vi "loop_config.vi"() -> ()   [LabVIEW 2017]
panel:
  in  "stop":bool
  out "error out":errorcluster
  in  "Read (TRUE)":bool
  in  "In":u8=22 format="%.0x"
  in  "Address":u32=2305 format="%x"
  out "Out":u8=22 format="%.0x"
  in  "address":string="192.168.10.20"
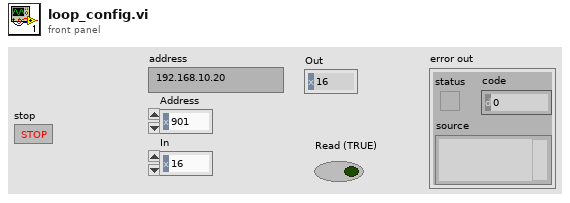
[diagram p1: front panel]
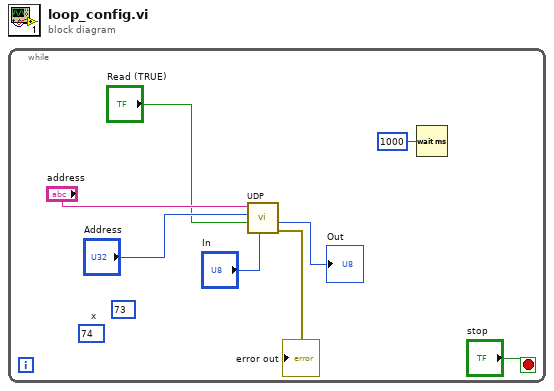
[diagram p0: block diagram]
diagram:
  n1 = while {
    stop <- "stop" stop-if-true
    (unwired) u32 73 ("Address")
    (unwired) u16 74  # x
    n2 = call "UDP.vi"("In"="In", "Read (TRUE)"="Read (TRUE)", "Address"="Address", "IP address"="address") -> ("error out"=→"error out":errorcluster, "Out"=→"Out":u8)  [unwired: 4 in, 1 out]
    n3 = Wait (ms)(milliseconds to wait=u32 1000) -> ()  [unwired: 1 out]
  }
